vi "Autonomous Independent.vi"() -> ()   [LabVIEW 2016]
doc: "This VI is called when autonomous begins, and will automatically be terminated when autonomous ends. You can carry out timed or sensor driven robot movement independently without needing to return to the caller."
uses:
  <vilib>/Rock Robotics/WPI/Utilities/WPI_GetSetVariantRefNum.vi
  <vilib>/Rock Robotics/WPI/RobotDrive/WPI_RobotDriveArcadeDrive_Standard(NoSaturation).vi
  <vilib>/Rock Robotics/Network Tables/SD Read Number.vi
  <vilib>/Rock Robotics/WPI/Solenoid/Deprecated/WPI_SolenoidSetBool.vi
panel:
  out "Current Movement, for debugging":T1 {"Y Joystick Value" scale=1.0..-1.0; "X Joystick Value" scale=-1.0..1.0}
  in  "Array of robot movements":T2(array[cluster]) {"Y Joystick Value" scale=1.0..-1.0; "X Joystick Value" scale=-1.0..1.0}
  # "Be sure to right-click and choose Data Operations>>Make Current Value default if you want to save the array values with the VI"
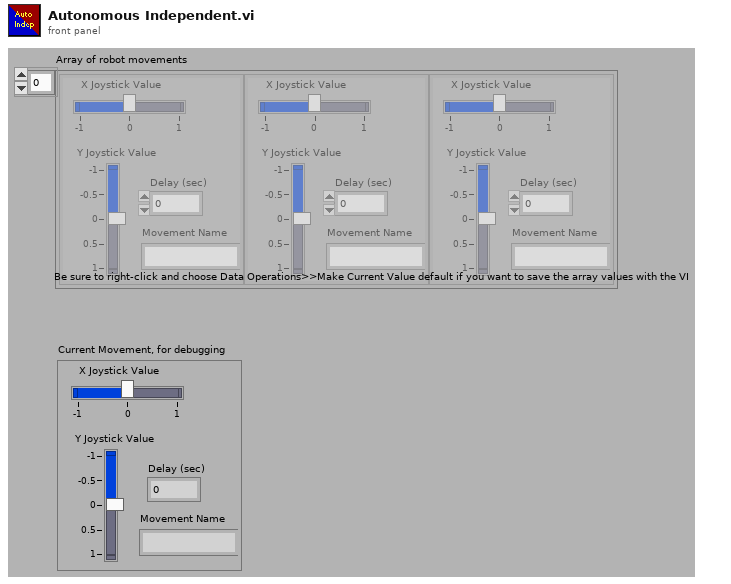
[diagram p1: front panel]
types:
  T1 = cluster{"X Joystick Value":dbl, "Y Joystick Value":dbl, "Delay (sec)":dbl, "Movement Name":string}
  T2 = cluster{"X Joystick Value":dbl, "Y Joystick Value":dbl, "Delay (sec)":dbl, "Movement Name":string}[]
  T3 = typedef "WPI_MotorControlDeviceRef.ctl" = cluster{"DeviceStatus":errorcluster, "Type":T4, "PWM":cluster{"PWM Channel":T5, "DeadBand":T6}, "CAN":cluster{"Device Number":u8, "SetOutput VI Ref":variant, "GetOutput VI Ref":variant, "Enable VI Ref":variant, "Disable VI Ref":variant, "Data":variant}, "Invert":bool}
  T4 = typedef "WPI_MotorControlType.ctl" = enum16{"PWM", "CAN"}
  T5 = typedef "FPGA_DIOPWMChannel.ctl" = enum8{"PWM 0", "PWM 1", "PWM 2", "PWM 3", "PWM 4", "PWM 5", "PWM 6", "PWM 7", "PWM 8", "PWM 9", "PWM MXP 0", "PWM MXP 1", "PWM MXP 2", "PWM MXP 3", "PWM MXP 4", "PWM MXP 5", "PWM MXP 6", "PWM MXP 7", "PWM MXP 8", "PWM MXP 9", "Invalid"}
  T6 = typedef "WPI_PWMDeadband.ctl" = cluster{"Name":string, "maxPositivePwm":i32, "minPositivePwm":i32, "centerPwm":i32, "maxNegativePwm":i32, "minNegativePwm":i32, "angularRange":u16}
  T7 = typedef "WPI_SolenoidDevRef.ctl" = cluster{"DevStatus":errorcluster, "Pneumatics Control Module":u8, "Forward Solenoid Channel":T8, "Reverse Solenoid Channel":T8}
  T8 = typedef "WPI_SolenoidChannel.ctl" = enum8{"Solenoid 0", "Solenoid 1", "Solenoid 2", "Solenoid 3", "Solenoid 4", "Solenoid 5", "Solenoid 6", "Solenoid 7", "Invalid"}
  T9 = typedef "WPI_RobotDriveDevRef.ctl" = cluster{"DevStatus":errorcluster, "Motors[]":T3[], "Square Inputs":bool, "Max Output":dbl}
  T10 = typedef "WPI_JoystickDevRef.ctl" = cluster{"Device":T11}
  T11 = typedef "WPI_JoystickDeviceEnum.ctl" = enum16{"USB 0", "USB 1", "USB 2", "USB 3", "USB 4", "USB 5"}
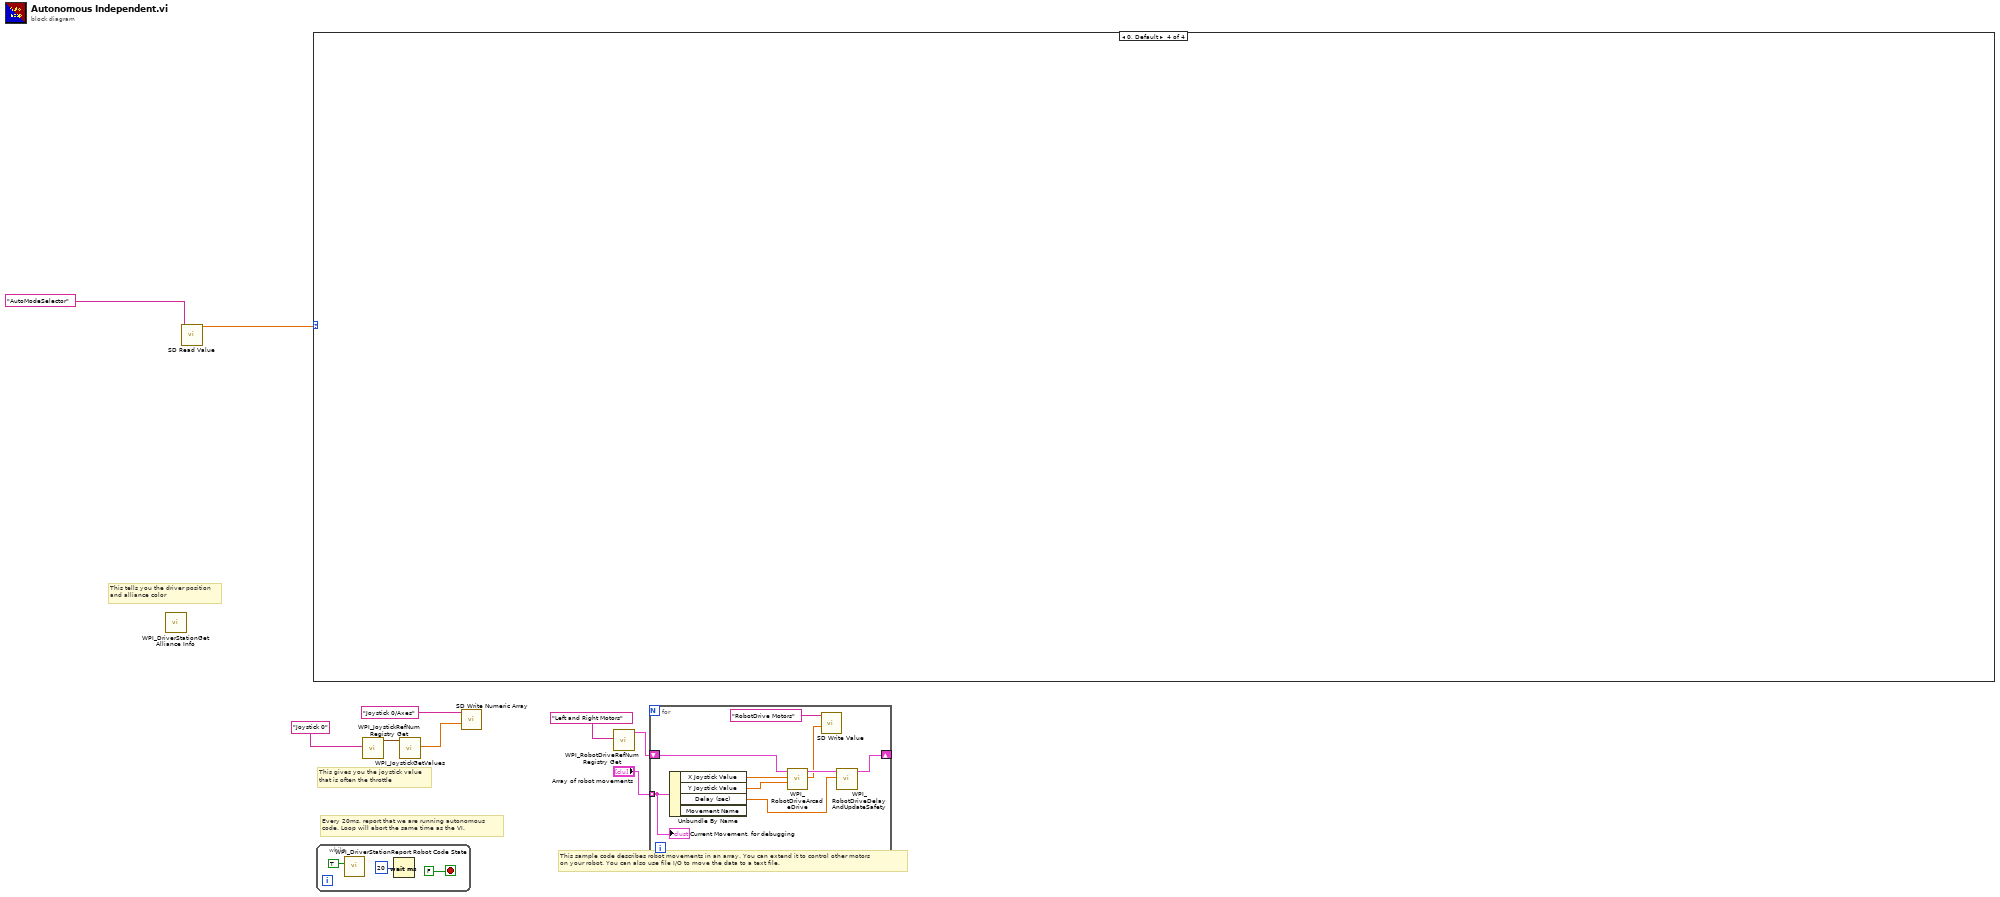
[diagram p0: block diagram]
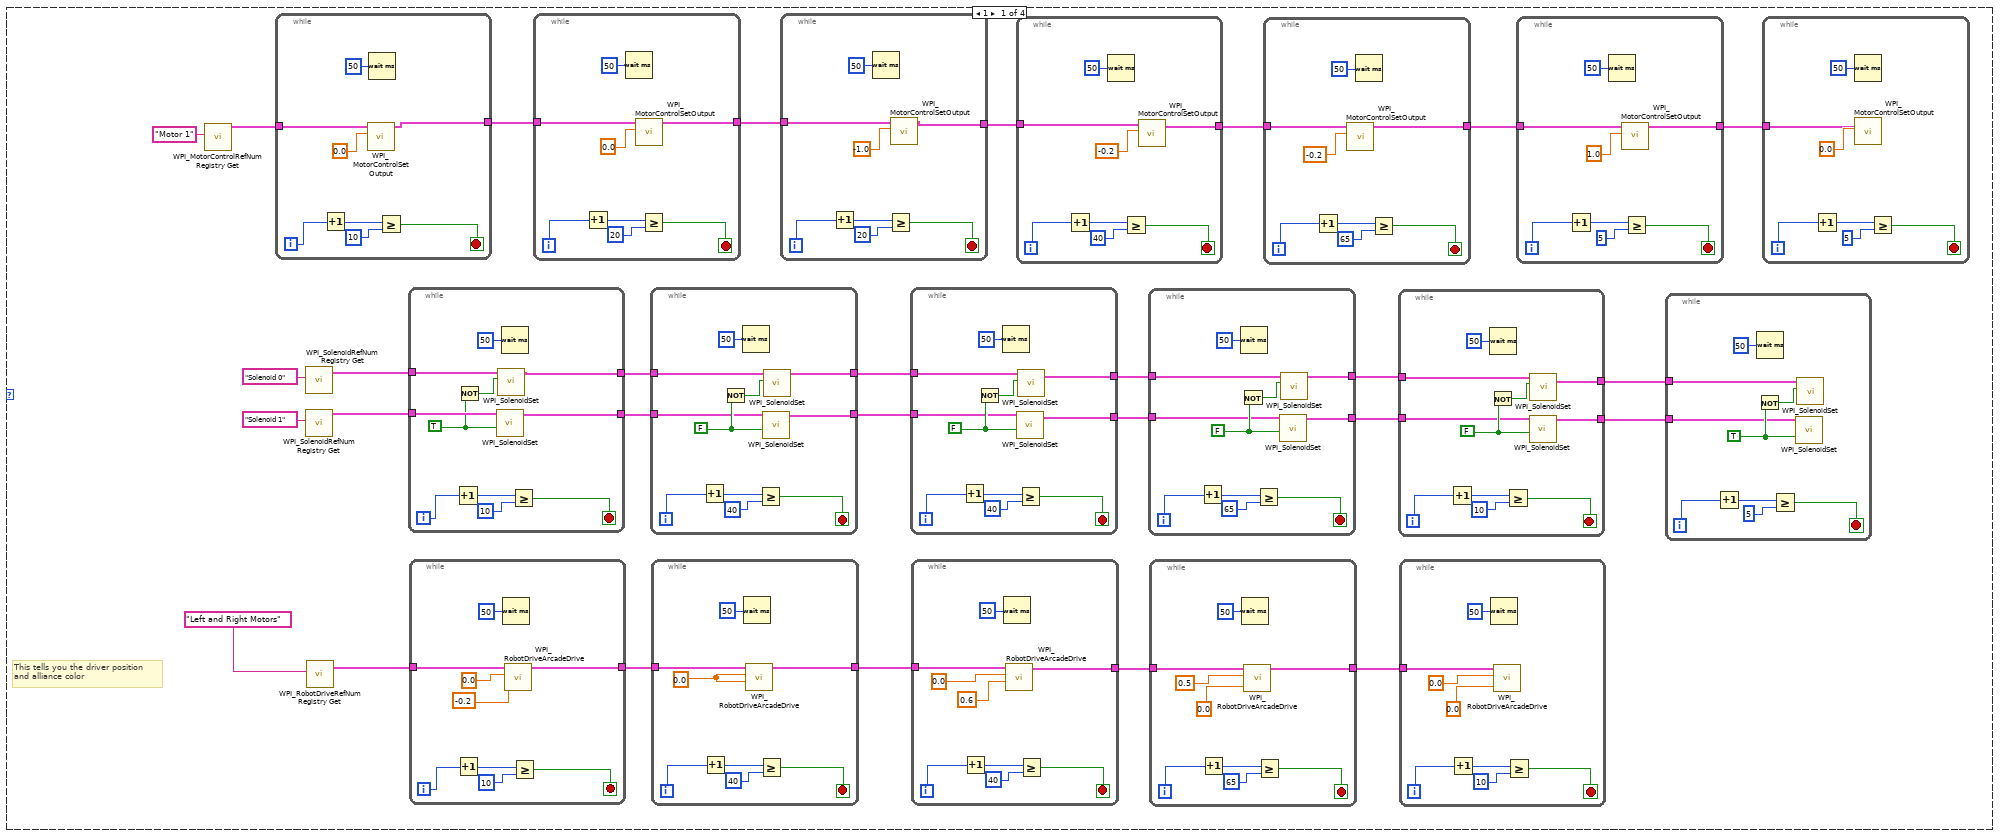
[diagram p2: hidden frame]
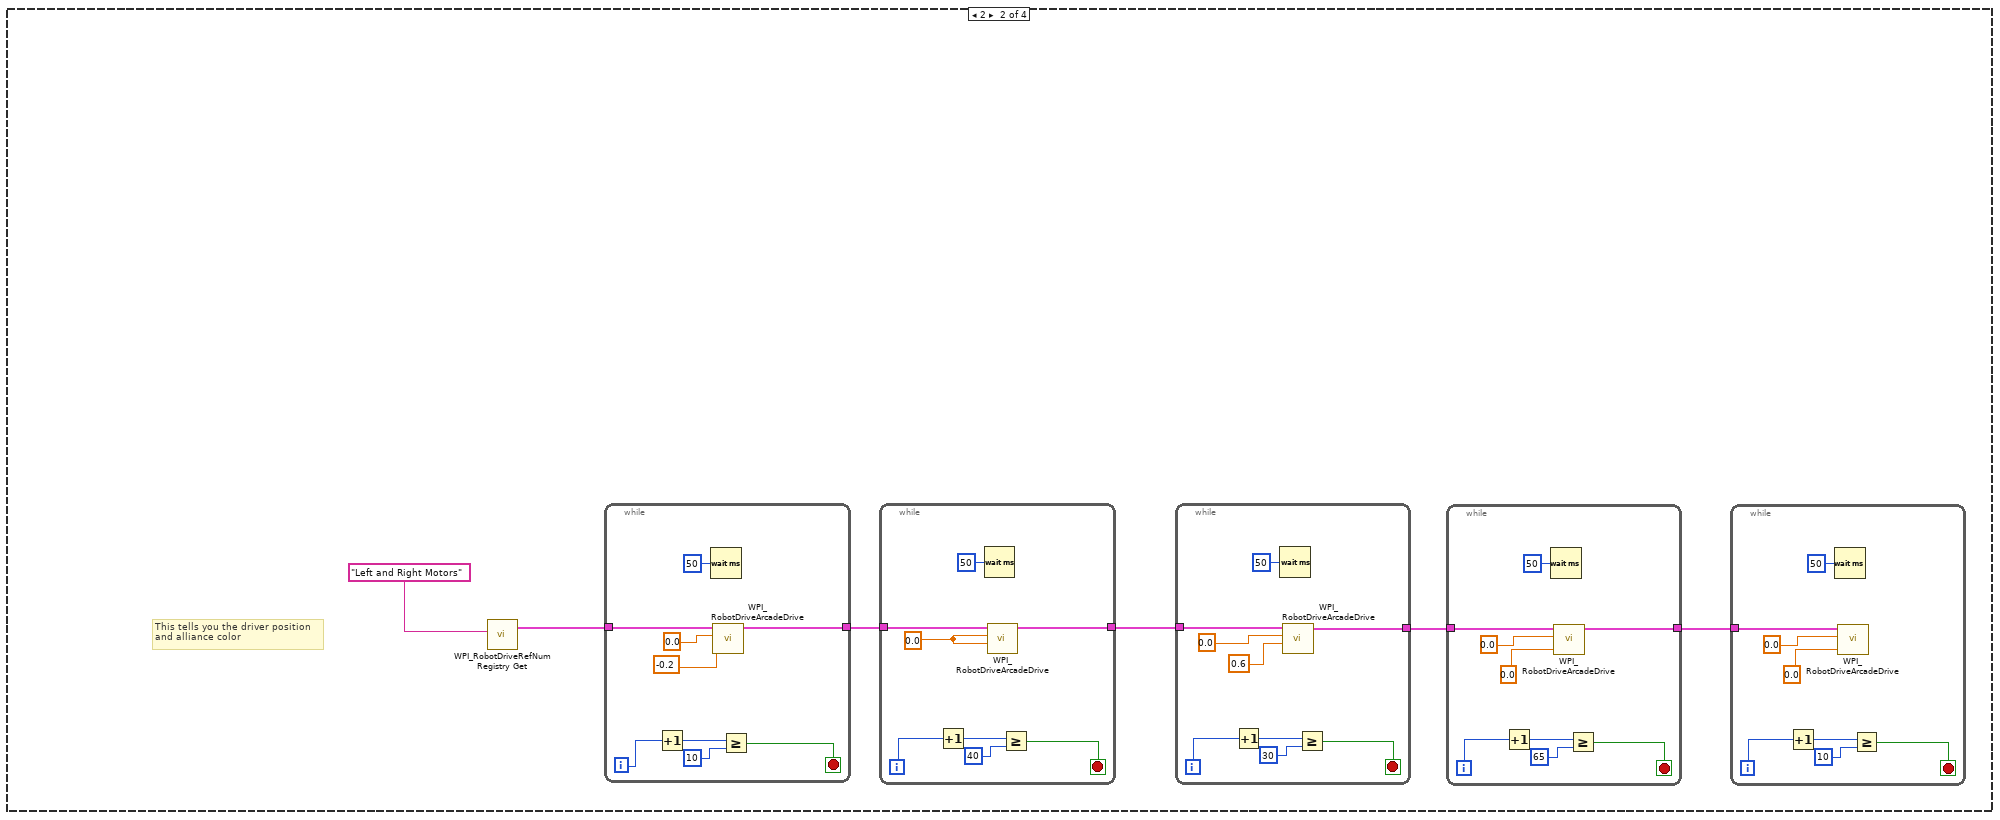
[diagram p3: hidden frame]
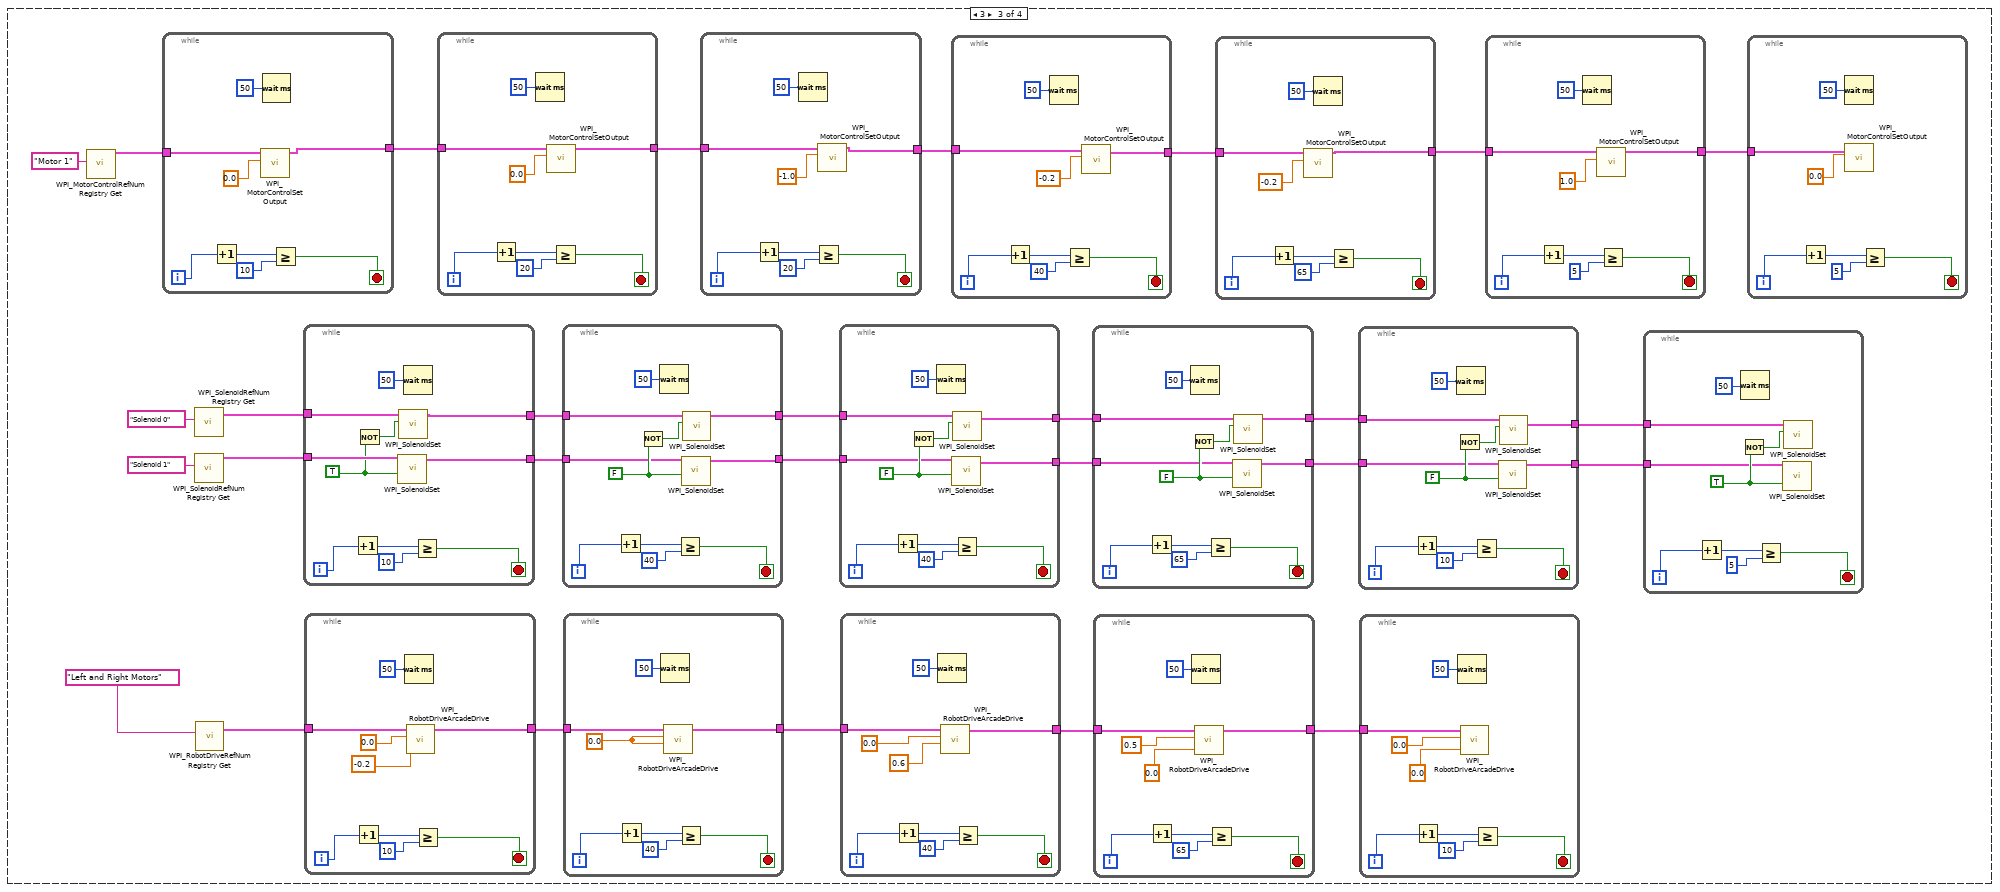
[diagram p4: hidden frame]
diagram:
  # "This tells you the driver position\nand alliance color"
  # "This sample code describes robot movements in an array. You can extend it to control other motors\non your robot. You can also use file I/O to move the data to a text file."
  # "Every 20ms, report that we are running autonomous\ncode. Loop will abort the same time as the VI."
  # "This gives you the joystick value\nthat is often the throttle"
  n1 = call <vilib>:"WPI_DriverStationGet Alliance Info.vi"() -> ()  [unwired: 12 out]
  n2 = call-poly <vilib>:"SD Read Value.vi"("Name"="AutoModeSelector") -> ("Numeric"=w2:dbl)  [unwired: 8 in, 2 out]
  n3 = case shown="0, Default" w2 {
    frame 1 {
      # "This tells you the driver position\nand alliance color"
      n4 = call <vilib>:"WPI_MotorControlRefNum Registry Get.vi"("refnum name"="Motor 1") -> ("MotorControlDevRef"=w18:T3)  [unwired: 9 in, 1 out]
      n5 = while {
        tunnel: w18 -> [w115]
        tunnel: [w113] -> w17
        i -> [w120]
        stop <- w116 stop-if-true
        n6 = Increment(x=w120) -> (x+1=w119:i32)
        n7 = call <vilib>:"WPI_MotorControlSetOutput.vi"("Output"=0.0, "MotorControlDevRef"=w115) -> ("MotorControlDevRef"=w113:T3)  [unwired: 7 in, 2 out]
        n8 = Wait (ms)(milliseconds to wait=u32 50) -> ()  [unwired: 1 out]
        n9 = Greater Or Equal?(x=w119, y=10) -> (x >= y?=w116:bool)
      }
      n10 = call <vilib>:"WPI_SolenoidRefNum Registry Get.vi"("refnum name"="Solenoid 0") -> ("SolenoidDevRef"=w30:T7)  [unwired: 9 in, 1 out]
      n11 = call <vilib>:"WPI_SolenoidRefNum Registry Get.vi"("refnum name"="Solenoid 1") -> ("SolenoidDevRef"=w29:T7)  [unwired: 9 in, 1 out]
      n12 = call <vilib>:"WPI_RobotDriveRefNum Registry Get.vi"("refnum name"="Left and Right Motors") -> ("RobotDriveDevRef"=w36:T9)  [unwired: 9 in, 1 out]
      n13 = while {
        tunnel: w30 -> [w159]
        tunnel: w29 -> [w158]
        tunnel: [w155] -> w28
        tunnel: [w154] -> w27
        i -> [w164]
        stop <- w160 stop-if-true
        w157 = TRUE
        n14 = Increment(x=w164) -> (x+1=w163:i32)
        n15 = Not(x=w157) -> (.not. x?=w156:bool)
        n16 = call-poly <vilib>:"WPI_SolenoidSet.vi"("Value"=w157, "SolenoidDevRef"=w158) -> ("SolenoidDevRef"=w154:T7)  [unwired: 8 in, 1 out]
        n17 = call-poly <vilib>:"WPI_SolenoidSet.vi"("Value"=w156, "SolenoidDevRef"=w159) -> ("SolenoidDevRef"=w155:T7)  [unwired: 8 in, 1 out]
        n18 = Wait (ms)(milliseconds to wait=u32 50) -> ()  [unwired: 1 out]
        n19 = Greater Or Equal?(x=w163, y=10) -> (x >= y?=w160:bool)
      }
      n20 = while {
        tunnel: w36 -> [w199]
        tunnel: [w192] -> w35
        i -> [w197]
        stop <- w193 stop-if-true
        n21 = Increment(x=w197) -> (x+1=w196:i32)
        n22 = Wait (ms)(milliseconds to wait=u32 50) -> ()  [unwired: 1 out]
        n23 = call-poly <vilib>:"WPI_RobotDriveArcadeDrive.vi"("Y axis value"=-0.2, "X axis value"=0.0, "RobotDriveDevRef"=w199) -> ("RobotDriveDevRef"=w192:T9)  [unwired: 6 in, 2 out]
        n24 = Greater Or Equal?(x=w196, y=10) -> (x >= y?=w193:bool)
      }
      n25 = while {
        tunnel: w17 -> [w106]
        tunnel: [w105] -> w16
        i -> [w108]
        stop <- w109 stop-if-true
        n26 = Increment(x=w108) -> (x+1=w111:i32)
        n27 = Wait (ms)(milliseconds to wait=u32 50) -> ()  [unwired: 1 out]
        n28 = call <vilib>:"WPI_MotorControlSetOutput.vi"("Output"=0.0, "MotorControlDevRef"=w106) -> ("MotorControlDevRef"=w105:T3)  [unwired: 7 in, 2 out]
        n29 = Greater Or Equal?(x=w111, y=20) -> (x >= y?=w109:bool)
      }
      n30 = while {
        tunnel: w28 -> [w146]
        tunnel: w27 -> [w145]
        tunnel: [w144] -> w26
        tunnel: [w143] -> w25
        i -> [w149]
        stop <- w150 stop-if-true
        w148 = FALSE
        n31 = Increment(x=w149) -> (x+1=w152:i32)
        n32 = Not(x=w148) -> (.not. x?=w147:bool)
        n33 = Wait (ms)(milliseconds to wait=u32 50) -> ()  [unwired: 1 out]
        n34 = Greater Or Equal?(x=w152, y=40) -> (x >= y?=w150:bool)
        n35 = call-poly <vilib>:"WPI_SolenoidSet.vi"("Value"=w148, "SolenoidDevRef"=w145) -> ("SolenoidDevRef"=w143:T7)  [unwired: 8 in, 1 out]
        n36 = call-poly <vilib>:"WPI_SolenoidSet.vi"("Value"=w147, "SolenoidDevRef"=w146) -> ("SolenoidDevRef"=w144:T7)  [unwired: 8 in, 1 out]
      }
      n37 = while {
        tunnel: w35 -> [w190]
        tunnel: [w183] -> w34
        i -> [w184]
        stop <- w185 stop-if-true
        w189 = 0.0 ("X axis value")
        n38 = Increment(x=w184) -> (x+1=w187:i32)
        n39 = Wait (ms)(milliseconds to wait=u32 50) -> ()  [unwired: 1 out]
        n40 = call-poly <vilib>:"WPI_RobotDriveArcadeDrive.vi"("Y axis value"=w189, "X axis value"=w189, "RobotDriveDevRef"=w190) -> ("RobotDriveDevRef"=w183:T9)  [unwired: 6 in, 2 out]
        n41 = Greater Or Equal?(x=w187, y=40) -> (x >= y?=w185:bool)
      }
      n42 = while {
        tunnel: w16 -> [w98]
        tunnel: [w97] -> w15
        i -> [w100]
        stop <- w101 stop-if-true
        n43 = Increment(x=w100) -> (x+1=w103:i32)
        n44 = Wait (ms)(milliseconds to wait=u32 50) -> ()  [unwired: 1 out]
        n45 = Greater Or Equal?(x=w103, y=20) -> (x >= y?=w101:bool)
        n46 = call <vilib>:"WPI_MotorControlSetOutput.vi"("Output"=-1.0, "MotorControlDevRef"=w98) -> ("MotorControlDevRef"=w97:T3)  [unwired: 7 in, 2 out]
      }
      n47 = while {
        tunnel: w26 -> [w135]
        tunnel: w25 -> [w134]
        tunnel: [w133] -> w23
        tunnel: [w132] -> w22
        i -> [w138]
        stop <- w139 stop-if-true
        w137 = FALSE
        n48 = Increment(x=w138) -> (x+1=w141:i32)
        n49 = Not(x=w137) -> (.not. x?=w136:bool)
        n50 = Wait (ms)(milliseconds to wait=u32 50) -> ()  [unwired: 1 out]
        n51 = call-poly <vilib>:"WPI_SolenoidSet.vi"("Value"=w137, "SolenoidDevRef"=w134) -> ("SolenoidDevRef"=w132:T7)  [unwired: 8 in, 1 out]
        n52 = call-poly <vilib>:"WPI_SolenoidSet.vi"("Value"=w136, "SolenoidDevRef"=w135) -> ("SolenoidDevRef"=w133:T7)  [unwired: 8 in, 1 out]
        n53 = Greater Or Equal?(x=w141, y=40) -> (x >= y?=w139:bool)
      }
      n54 = while {
        tunnel: w34 -> [w182]
        tunnel: [w174] -> w33
        i -> [w177]
        stop <- w178 stop-if-true
        n55 = Increment(x=w177) -> (x+1=w180:i32)
        n56 = Wait (ms)(milliseconds to wait=u32 50) -> ()  [unwired: 1 out]
        n57 = call-poly <vilib>:"WPI_RobotDriveArcadeDrive.vi"("Y axis value"=0.6, "X axis value"=0.0, "RobotDriveDevRef"=w182) -> ("RobotDriveDevRef"=w174:T9)  [unwired: 6 in, 2 out]
        n58 = Greater Or Equal?(x=w180, y=40) -> (x >= y?=w178:bool)
      }
      n59 = while {
        tunnel: w15 -> [w90]
        tunnel: [w89] -> w14
        i -> [w92]
        stop <- w93 stop-if-true
        n60 = Increment(x=w92) -> (x+1=w95:i32)
        n61 = Wait (ms)(milliseconds to wait=u32 50) -> ()  [unwired: 1 out]
        n62 = Greater Or Equal?(x=w95, y=40) -> (x >= y?=w93:bool)
        n63 = call <vilib>:"WPI_MotorControlSetOutput.vi"("Output"=-0.2, "MotorControlDevRef"=w90) -> ("MotorControlDevRef"=w89:T3)  [unwired: 7 in, 2 out]
      }
      n64 = while {
        tunnel: w23 -> [w124]
        tunnel: w22 -> [w123]
        tunnel: [w122] -> w21
        tunnel: [w121] -> w20
        i -> [w127]
        stop <- w128 stop-if-true
        w126 = FALSE
        n65 = Increment(x=w127) -> (x+1=w130:i32)
        n66 = Not(x=w126) -> (.not. x?=w125:bool)
        n67 = Wait (ms)(milliseconds to wait=u32 50) -> ()  [unwired: 1 out]
        n68 = Greater Or Equal?(x=w130, y=65) -> (x >= y?=w128:bool)
        n69 = call-poly <vilib>:"WPI_SolenoidSet.vi"("Value"=w126, "SolenoidDevRef"=w123) -> ("SolenoidDevRef"=w121:T7)  [unwired: 8 in, 1 out]
        n70 = call-poly <vilib>:"WPI_SolenoidSet.vi"("Value"=w125, "SolenoidDevRef"=w124) -> ("SolenoidDevRef"=w122:T7)  [unwired: 8 in, 1 out]
      }
      n71 = while {
        tunnel: w33 -> [w173]
        tunnel: [w165] -> w24
        i -> [w167]
        stop <- w168 stop-if-true
        n72 = Increment(x=w167) -> (x+1=w170:i32)
        n73 = Wait (ms)(milliseconds to wait=u32 50) -> ()  [unwired: 1 out]
        n74 = call-poly <vilib>:"WPI_RobotDriveArcadeDrive.vi"("Y axis value"=0.0 ("X axis value"), "X axis value"=0.5, "RobotDriveDevRef"=w173) -> ("RobotDriveDevRef"=w165:T9)  [unwired: 6 in, 2 out]
        n75 = Greater Or Equal?(x=w170, y=65) -> (x >= y?=w168:bool)
      }
      n76 = while {
        tunnel: w14 -> [w63]
        tunnel: [w62] -> w13
        i -> [w65]
        stop <- w66 stop-if-true
        n77 = Increment(x=w65) -> (x+1=w68:i32)
        n78 = call <vilib>:"WPI_MotorControlSetOutput.vi"("Output"=-0.2, "MotorControlDevRef"=w63) -> ("MotorControlDevRef"=w62:T3)  [unwired: 7 in, 2 out]
        n79 = Wait (ms)(milliseconds to wait=u32 50) -> ()  [unwired: 1 out]
        n80 = Greater Or Equal?(x=w68, y=65) -> (x >= y?=w66:bool)
      }
      n81 = while {
        tunnel: w21 -> [w73]
        tunnel: w20 -> [w72]
        tunnel: [w71] -> w11
        tunnel: [w70] -> w10
        i -> [w76]
        stop <- w77 stop-if-true
        w75 = FALSE
        n82 = Increment(x=w76) -> (x+1=w79:i32)
        n83 = Not(x=w75) -> (.not. x?=w74:bool)
        n84 = Wait (ms)(milliseconds to wait=u32 50) -> ()  [unwired: 1 out]
        n85 = Greater Or Equal?(x=w79, y=10) -> (x >= y?=w77:bool)
        n86 = call-poly <vilib>:"WPI_SolenoidSet.vi"("Value"=w75, "SolenoidDevRef"=w72) -> ("SolenoidDevRef"=w70:T7)  [unwired: 8 in, 1 out]
        n87 = call-poly <vilib>:"WPI_SolenoidSet.vi"("Value"=w74, "SolenoidDevRef"=w73) -> ("SolenoidDevRef"=w71:T7)  [unwired: 8 in, 1 out]
      }
      n88 = while {
        tunnel: w24 -> [w88]
        i -> [w82]
        stop <- w83 stop-if-true
        n89 = Increment(x=w82) -> (x+1=w85:i32)
        n90 = Wait (ms)(milliseconds to wait=u32 50) -> ()  [unwired: 1 out]
        n91 = call-poly <vilib>:"WPI_RobotDriveArcadeDrive.vi"("Y axis value"=0.0 ("X axis value"), "X axis value"=0.0, "RobotDriveDevRef"=w88) -> ()  [unwired: 6 in, 3 out]
        n92 = Greater Or Equal?(x=w85, y=10) -> (x >= y?=w83:bool)
      }
      n93 = while {
        tunnel: w13 -> [w55]
        tunnel: [w54] -> w12
        i -> [w57]
        stop <- w58 stop-if-true
        n94 = Increment(x=w57) -> (x+1=w60:i32)
        n95 = Wait (ms)(milliseconds to wait=u32 50) -> ()  [unwired: 1 out]
        n96 = call <vilib>:"WPI_MotorControlSetOutput.vi"("Output"=1.0, "MotorControlDevRef"=w55) -> ("MotorControlDevRef"=w54:T3)  [unwired: 7 in, 2 out]
        n97 = Greater Or Equal?(x=w60, y=5) -> (x >= y?=w58:bool)
      }
      n98 = while {
        tunnel: w11 -> [w39]
        tunnel: w10 -> [w38]
        i -> [w42]
        stop <- w43 stop-if-true
        w41 = TRUE
        n99 = Increment(x=w42) -> (x+1=w45:i32)
        n100 = Not(x=w41) -> (.not. x?=w40:bool)
        n101 = Wait (ms)(milliseconds to wait=u32 50) -> ()  [unwired: 1 out]
        n102 = Greater Or Equal?(x=w45, y=5) -> (x >= y?=w43:bool)
        n103 = call-poly <vilib>:"WPI_SolenoidSet.vi"("Value"=w41, "SolenoidDevRef"=w38) -> ()  [unwired: 8 in, 2 out]
        n104 = call-poly <vilib>:"WPI_SolenoidSet.vi"("Value"=w40, "SolenoidDevRef"=w39) -> ()  [unwired: 8 in, 2 out]
      }
      n105 = while {
        tunnel: w12 -> [w47]
        i -> [w49]
        stop <- w50 stop-if-true
        n106 = Increment(x=w49) -> (x+1=w52:i32)
        n107 = Wait (ms)(milliseconds to wait=u32 50) -> ()  [unwired: 1 out]
        n108 = call <vilib>:"WPI_MotorControlSetOutput.vi"("Output"=0.0, "MotorControlDevRef"=w47) -> ()  [unwired: 7 in, 3 out]
        n109 = Greater Or Equal?(x=w52, y=5) -> (x >= y?=w50:bool)
      }
    }
    frame 2 {
      # "This tells you the driver position\nand alliance color"
      n110 = call <vilib>:"WPI_RobotDriveRefNum Registry Get.vi"("refnum name"="Left and Right Motors") -> ("RobotDriveDevRef"=w204:T9)  [unwired: 9 in, 1 out]
      n111 = while {
        tunnel: w204 -> [w248]
        tunnel: [w241] -> w203
        i -> [w246]
        stop <- w242 stop-if-true
        n112 = Increment(x=w246) -> (x+1=w245:i32)
        n113 = Wait (ms)(milliseconds to wait=u32 50) -> ()  [unwired: 1 out]
        n114 = call-poly <vilib>:"WPI_RobotDriveArcadeDrive.vi"("Y axis value"=-0.2, "X axis value"=0.0, "RobotDriveDevRef"=w248) -> ("RobotDriveDevRef"=w241:T9)  [unwired: 6 in, 2 out]
        n115 = Greater Or Equal?(x=w245, y=10) -> (x >= y?=w242:bool)
      }
      n116 = while {
        tunnel: w203 -> [w239]
        tunnel: [w232] -> w202
        i -> [w233]
        stop <- w234 stop-if-true
        w238 = 0.0 ("X axis value")
        n117 = Increment(x=w233) -> (x+1=w236:i32)
        n118 = Wait (ms)(milliseconds to wait=u32 50) -> ()  [unwired: 1 out]
        n119 = call-poly <vilib>:"WPI_RobotDriveArcadeDrive.vi"("Y axis value"=w238, "X axis value"=w238, "RobotDriveDevRef"=w239) -> ("RobotDriveDevRef"=w232:T9)  [unwired: 6 in, 2 out]
        n120 = Greater Or Equal?(x=w236, y=40) -> (x >= y?=w234:bool)
      }
      n121 = while {
        tunnel: w202 -> [w231]
        tunnel: [w223] -> w201
        i -> [w226]
        stop <- w227 stop-if-true
        n122 = Increment(x=w226) -> (x+1=w229:i32)
        n123 = Wait (ms)(milliseconds to wait=u32 50) -> ()  [unwired: 1 out]
        n124 = call-poly <vilib>:"WPI_RobotDriveArcadeDrive.vi"("Y axis value"=0.6, "X axis value"=0.0, "RobotDriveDevRef"=w231) -> ("RobotDriveDevRef"=w223:T9)  [unwired: 6 in, 2 out]
        n125 = Greater Or Equal?(x=w229, y=30) -> (x >= y?=w227:bool)
      }
      n126 = while {
        tunnel: w201 -> [w222]
        tunnel: [w214] -> w200
        i -> [w216]
        stop <- w217 stop-if-true
        n127 = Increment(x=w216) -> (x+1=w219:i32)
        n128 = Wait (ms)(milliseconds to wait=u32 50) -> ()  [unwired: 1 out]
        n129 = call-poly <vilib>:"WPI_RobotDriveArcadeDrive.vi"("Y axis value"=0.0 ("X axis value"), "X axis value"=0.0, "RobotDriveDevRef"=w222) -> ("RobotDriveDevRef"=w214:T9)  [unwired: 6 in, 2 out]
        n130 = Greater Or Equal?(x=w219, y=65) -> (x >= y?=w217:bool)
      }
      n131 = while {
        tunnel: w200 -> [w213]
        i -> [w207]
        stop <- w208 stop-if-true
        n132 = Increment(x=w207) -> (x+1=w210:i32)
        n133 = Wait (ms)(milliseconds to wait=u32 50) -> ()  [unwired: 1 out]
        n134 = call-poly <vilib>:"WPI_RobotDriveArcadeDrive.vi"("Y axis value"=0.0 ("X axis value"), "X axis value"=0.0, "RobotDriveDevRef"=w213) -> ()  [unwired: 6 in, 3 out]
        n135 = Greater Or Equal?(x=w210, y=10) -> (x >= y?=w208:bool)
      }
    }
    frame 3 {
      n136 = call <vilib>:"WPI_MotorControlRefNum Registry Get.vi"("refnum name"="Motor 1") -> ("MotorControlDevRef"=w257:T3)  [unwired: 9 in, 1 out]
      n137 = while {
        tunnel: w257 -> [w354]
        tunnel: [w352] -> w256
        i -> [w359]
        stop <- w355 stop-if-true
        n138 = Increment(x=w359) -> (x+1=w358:i32)
        n139 = call <vilib>:"WPI_MotorControlSetOutput.vi"("Output"=0.0, "MotorControlDevRef"=w354) -> ("MotorControlDevRef"=w352:T3)  [unwired: 7 in, 2 out]
        n140 = Wait (ms)(milliseconds to wait=u32 50) -> ()  [unwired: 1 out]
        n141 = Greater Or Equal?(x=w358, y=10) -> (x >= y?=w355:bool)
      }
      n142 = call <vilib>:"WPI_SolenoidRefNum Registry Get.vi"("refnum name"="Solenoid 0") -> ("SolenoidDevRef"=w269:T7)  [unwired: 9 in, 1 out]
      n143 = call <vilib>:"WPI_SolenoidRefNum Registry Get.vi"("refnum name"="Solenoid 1") -> ("SolenoidDevRef"=w268:T7)  [unwired: 9 in, 1 out]
      n144 = call <vilib>:"WPI_RobotDriveRefNum Registry Get.vi"("refnum name"="Left and Right Motors") -> ("RobotDriveDevRef"=w275:T9)  [unwired: 9 in, 1 out]
      n145 = while {
        tunnel: w269 -> [w398]
        tunnel: w268 -> [w397]
        tunnel: [w394] -> w267
        tunnel: [w393] -> w266
        i -> [w403]
        stop <- w399 stop-if-true
        w396 = TRUE
        n146 = Increment(x=w403) -> (x+1=w402:i32)
        n147 = Not(x=w396) -> (.not. x?=w395:bool)
        n148 = call-poly <vilib>:"WPI_SolenoidSet.vi"("Value"=w396, "SolenoidDevRef"=w397) -> ("SolenoidDevRef"=w393:T7)  [unwired: 8 in, 1 out]
        n149 = call-poly <vilib>:"WPI_SolenoidSet.vi"("Value"=w395, "SolenoidDevRef"=w398) -> ("SolenoidDevRef"=w394:T7)  [unwired: 8 in, 1 out]
        n150 = Wait (ms)(milliseconds to wait=u32 50) -> ()  [unwired: 1 out]
        n151 = Greater Or Equal?(x=w402, y=10) -> (x >= y?=w399:bool)
      }
      n152 = while {
        tunnel: w275 -> [w438]
        tunnel: [w431] -> w274
        i -> [w436]
        stop <- w432 stop-if-true
        n153 = Increment(x=w436) -> (x+1=w435:i32)
        n154 = Wait (ms)(milliseconds to wait=u32 50) -> ()  [unwired: 1 out]
        n155 = call-poly <vilib>:"WPI_RobotDriveArcadeDrive.vi"("Y axis value"=-0.2, "X axis value"=0.0, "RobotDriveDevRef"=w438) -> ("RobotDriveDevRef"=w431:T9)  [unwired: 6 in, 2 out]
        n156 = Greater Or Equal?(x=w435, y=10) -> (x >= y?=w432:bool)
      }
      n157 = while {
        tunnel: w256 -> [w345]
        tunnel: [w344] -> w255
        i -> [w347]
        stop <- w348 stop-if-true
        n158 = Increment(x=w347) -> (x+1=w350:i32)
        n159 = Wait (ms)(milliseconds to wait=u32 50) -> ()  [unwired: 1 out]
        n160 = call <vilib>:"WPI_MotorControlSetOutput.vi"("Output"=0.0, "MotorControlDevRef"=w345) -> ("MotorControlDevRef"=w344:T3)  [unwired: 7 in, 2 out]
        n161 = Greater Or Equal?(x=w350, y=20) -> (x >= y?=w348:bool)
      }
      n162 = while {
        tunnel: w267 -> [w385]
        tunnel: w266 -> [w384]
        tunnel: [w383] -> w265
        tunnel: [w382] -> w264
        i -> [w388]
        stop <- w389 stop-if-true
        w387 = FALSE
        n163 = Increment(x=w388) -> (x+1=w391:i32)
        n164 = Not(x=w387) -> (.not. x?=w386:bool)
        n165 = Wait (ms)(milliseconds to wait=u32 50) -> ()  [unwired: 1 out]
        n166 = Greater Or Equal?(x=w391, y=40) -> (x >= y?=w389:bool)
        n167 = call-poly <vilib>:"WPI_SolenoidSet.vi"("Value"=w387, "SolenoidDevRef"=w384) -> ("SolenoidDevRef"=w382:T7)  [unwired: 8 in, 1 out]
        n168 = call-poly <vilib>:"WPI_SolenoidSet.vi"("Value"=w386, "SolenoidDevRef"=w385) -> ("SolenoidDevRef"=w383:T7)  [unwired: 8 in, 1 out]
      }
      n169 = while {
        tunnel: w274 -> [w429]
        tunnel: [w422] -> w273
        i -> [w423]
        stop <- w424 stop-if-true
        w428 = 0.0 ("X axis value")
        n170 = Increment(x=w423) -> (x+1=w426:i32)
        n171 = Wait (ms)(milliseconds to wait=u32 50) -> ()  [unwired: 1 out]
        n172 = call-poly <vilib>:"WPI_RobotDriveArcadeDrive.vi"("Y axis value"=w428, "X axis value"=w428, "RobotDriveDevRef"=w429) -> ("RobotDriveDevRef"=w422:T9)  [unwired: 6 in, 2 out]
        n173 = Greater Or Equal?(x=w426, y=40) -> (x >= y?=w424:bool)
      }
      n174 = while {
        tunnel: w255 -> [w337]
        tunnel: [w336] -> w254
        i -> [w339]
        stop <- w340 stop-if-true
        n175 = Increment(x=w339) -> (x+1=w342:i32)
        n176 = Wait (ms)(milliseconds to wait=u32 50) -> ()  [unwired: 1 out]
        n177 = Greater Or Equal?(x=w342, y=20) -> (x >= y?=w340:bool)
        n178 = call <vilib>:"WPI_MotorControlSetOutput.vi"("Output"=-1.0, "MotorControlDevRef"=w337) -> ("MotorControlDevRef"=w336:T3)  [unwired: 7 in, 2 out]
      }
      n179 = while {
        tunnel: w265 -> [w374]
        tunnel: w264 -> [w373]
        tunnel: [w372] -> w262
        tunnel: [w371] -> w261
        i -> [w377]
        stop <- w378 stop-if-true
        w376 = FALSE
        n180 = Increment(x=w377) -> (x+1=w380:i32)
        n181 = Not(x=w376) -> (.not. x?=w375:bool)
        n182 = Wait (ms)(milliseconds to wait=u32 50) -> ()  [unwired: 1 out]
        n183 = call-poly <vilib>:"WPI_SolenoidSet.vi"("Value"=w376, "SolenoidDevRef"=w373) -> ("SolenoidDevRef"=w371:T7)  [unwired: 8 in, 1 out]
        n184 = call-poly <vilib>:"WPI_SolenoidSet.vi"("Value"=w375, "SolenoidDevRef"=w374) -> ("SolenoidDevRef"=w372:T7)  [unwired: 8 in, 1 out]
        n185 = Greater Or Equal?(x=w380, y=40) -> (x >= y?=w378:bool)
      }
      n186 = while {
        tunnel: w273 -> [w421]
        tunnel: [w413] -> w272
        i -> [w416]
        stop <- w417 stop-if-true
        n187 = Increment(x=w416) -> (x+1=w419:i32)
        n188 = Wait (ms)(milliseconds to wait=u32 50) -> ()  [unwired: 1 out]
        n189 = call-poly <vilib>:"WPI_RobotDriveArcadeDrive.vi"("Y axis value"=0.6, "X axis value"=0.0, "RobotDriveDevRef"=w421) -> ("RobotDriveDevRef"=w413:T9)  [unwired: 6 in, 2 out]
        n190 = Greater Or Equal?(x=w419, y=40) -> (x >= y?=w417:bool)
      }
      n191 = while {
        tunnel: w254 -> [w329]
        tunnel: [w328] -> w253
        i -> [w331]
        stop <- w332 stop-if-true
        n192 = Increment(x=w331) -> (x+1=w334:i32)
        n193 = Wait (ms)(milliseconds to wait=u32 50) -> ()  [unwired: 1 out]
        n194 = Greater Or Equal?(x=w334, y=40) -> (x >= y?=w332:bool)
        n195 = call <vilib>:"WPI_MotorControlSetOutput.vi"("Output"=-0.2, "MotorControlDevRef"=w329) -> ("MotorControlDevRef"=w328:T3)  [unwired: 7 in, 2 out]
      }
      n196 = while {
        tunnel: w262 -> [w363]
        tunnel: w261 -> [w362]
        tunnel: [w361] -> w260
        tunnel: [w360] -> w259
        i -> [w366]
        stop <- w367 stop-if-true
        w365 = FALSE
        n197 = Increment(x=w366) -> (x+1=w369:i32)
        n198 = Not(x=w365) -> (.not. x?=w364:bool)
        n199 = Wait (ms)(milliseconds to wait=u32 50) -> ()  [unwired: 1 out]
        n200 = Greater Or Equal?(x=w369, y=65) -> (x >= y?=w367:bool)
        n201 = call-poly <vilib>:"WPI_SolenoidSet.vi"("Value"=w365, "SolenoidDevRef"=w362) -> ("SolenoidDevRef"=w360:T7)  [unwired: 8 in, 1 out]
        n202 = call-poly <vilib>:"WPI_SolenoidSet.vi"("Value"=w364, "SolenoidDevRef"=w363) -> ("SolenoidDevRef"=w361:T7)  [unwired: 8 in, 1 out]
      }
      n203 = while {
        tunnel: w272 -> [w412]
        tunnel: [w404] -> w263
        i -> [w406]
        stop <- w407 stop-if-true
        n204 = Increment(x=w406) -> (x+1=w409:i32)
        n205 = Wait (ms)(milliseconds to wait=u32 50) -> ()  [unwired: 1 out]
        n206 = call-poly <vilib>:"WPI_RobotDriveArcadeDrive.vi"("Y axis value"=0.0 ("X axis value"), "X axis value"=0.5, "RobotDriveDevRef"=w412) -> ("RobotDriveDevRef"=w404:T9)  [unwired: 6 in, 2 out]
        n207 = Greater Or Equal?(x=w409, y=65) -> (x >= y?=w407:bool)
      }
      n208 = while {
        tunnel: w253 -> [w302]
        tunnel: [w301] -> w252
        i -> [w304]
        stop <- w305 stop-if-true
        n209 = Increment(x=w304) -> (x+1=w307:i32)
        n210 = call <vilib>:"WPI_MotorControlSetOutput.vi"("Output"=-0.2, "MotorControlDevRef"=w302) -> ("MotorControlDevRef"=w301:T3)  [unwired: 7 in, 2 out]
        n211 = Wait (ms)(milliseconds to wait=u32 50) -> ()  [unwired: 1 out]
        n212 = Greater Or Equal?(x=w307, y=65) -> (x >= y?=w305:bool)
      }
      n213 = while {
        tunnel: w260 -> [w312]
        tunnel: w259 -> [w311]
        tunnel: [w310] -> w250
        tunnel: [w309] -> w249
        i -> [w315]
        stop <- w316 stop-if-true
        w314 = FALSE
        n214 = Increment(x=w315) -> (x+1=w318:i32)
        n215 = Not(x=w314) -> (.not. x?=w313:bool)
        n216 = Wait (ms)(milliseconds to wait=u32 50) -> ()  [unwired: 1 out]
        n217 = Greater Or Equal?(x=w318, y=10) -> (x >= y?=w316:bool)
        n218 = call-poly <vilib>:"WPI_SolenoidSet.vi"("Value"=w314, "SolenoidDevRef"=w311) -> ("SolenoidDevRef"=w309:T7)  [unwired: 8 in, 1 out]
        n219 = call-poly <vilib>:"WPI_SolenoidSet.vi"("Value"=w313, "SolenoidDevRef"=w312) -> ("SolenoidDevRef"=w310:T7)  [unwired: 8 in, 1 out]
      }
      n220 = while {
        tunnel: w263 -> [w327]
        i -> [w321]
        stop <- w322 stop-if-true
        n221 = Increment(x=w321) -> (x+1=w324:i32)
        n222 = Wait (ms)(milliseconds to wait=u32 50) -> ()  [unwired: 1 out]
        n223 = call-poly <vilib>:"WPI_RobotDriveArcadeDrive.vi"("Y axis value"=0.0 ("X axis value"), "X axis value"=0.0, "RobotDriveDevRef"=w327) -> ()  [unwired: 6 in, 3 out]
        n224 = Greater Or Equal?(x=w324, y=10) -> (x >= y?=w322:bool)
      }
      n225 = while {
        tunnel: w252 -> [w294]
        tunnel: [w293] -> w251
        i -> [w296]
        stop <- w297 stop-if-true
        n226 = Increment(x=w296) -> (x+1=w299:i32)
        n227 = Wait (ms)(milliseconds to wait=u32 50) -> ()  [unwired: 1 out]
        n228 = call <vilib>:"WPI_MotorControlSetOutput.vi"("Output"=1.0, "MotorControlDevRef"=w294) -> ("MotorControlDevRef"=w293:T3)  [unwired: 7 in, 2 out]
        n229 = Greater Or Equal?(x=w299, y=5) -> (x >= y?=w297:bool)
      }
      n230 = while {
        tunnel: w250 -> [w278]
        tunnel: w249 -> [w277]
        i -> [w281]
        stop <- w282 stop-if-true
        w280 = TRUE
        n231 = Increment(x=w281) -> (x+1=w284:i32)
        n232 = Not(x=w280) -> (.not. x?=w279:bool)
        n233 = Wait (ms)(milliseconds to wait=u32 50) -> ()  [unwired: 1 out]
        n234 = Greater Or Equal?(x=w284, y=5) -> (x >= y?=w282:bool)
        n235 = call-poly <vilib>:"WPI_SolenoidSet.vi"("Value"=w280, "SolenoidDevRef"=w277) -> ()  [unwired: 8 in, 2 out]
        n236 = call-poly <vilib>:"WPI_SolenoidSet.vi"("Value"=w279, "SolenoidDevRef"=w278) -> ()  [unwired: 8 in, 2 out]
      }
      n237 = while {
        tunnel: w251 -> [w286]
        i -> [w288]
        stop <- w289 stop-if-true
        n238 = Increment(x=w288) -> (x+1=w291:i32)
        n239 = Wait (ms)(milliseconds to wait=u32 50) -> ()  [unwired: 1 out]
        n240 = call <vilib>:"WPI_MotorControlSetOutput.vi"("Output"=0.0, "MotorControlDevRef"=w286) -> ()  [unwired: 7 in, 3 out]
        n241 = Greater Or Equal?(x=w291, y=5) -> (x >= y?=w289:bool)
      }
    }
    frame 0, Default {
    }
  }
  n242 = while {
    stop <- FALSE stop-if-true
    n243 = call <vilib>:"WPI_DriverStationReport Robot Code State.vi"("Autonomous"=TRUE) -> ()  [unwired: 10 in, 1 out]
    n244 = Wait (ms)(milliseconds to wait=u32 20) -> ()  [unwired: 1 out]
  }
  n245 = call <vilib>:"WPI_JoystickRefNum Registry Get.vi"("refnum name"="Joystick 0") -> ("JoystickDevRef"=w8:T10)  [unwired: 1 in, 9 out]
  n246 = call <vilib>:"WPI_JoystickGetValues.vi"("JoystickDevRef"=w8) -> ("Axes"=w6:dbl[])  [unwired: 6 in, 4 out]
  n247 = call <vilib>:"SD Write Numeric Array.vi"("Numeric Array"=w6, "Name"="Joystick 0/Axes") -> ()  [unwired: 8 in, 2 out]
  n248 = call <vilib>:"WPI_RobotDriveRefNum Registry Get.vi"("refnum name"="Left and Right Motors") -> ("RobotDriveDevRef"=w4:T9)  [unwired: 1 in, 9 out]
  n249 = for {
    shift-right: [w447] -> _
    shift-left: w4 -> [w448]
    tunnel: "Array of robot movements" -> [w443] mode=indexing
    n250 = Unbundle By Name(w443) -> ("X Joystick Value"=w446:dbl, "Y Joystick Value"=w445:dbl, "Delay (sec)"=w444:dbl)  [unwired: 1 out]
    n251 = call-poly <vilib>:"WPI_RobotDriveArcadeDrive.vi"("Y axis value"=w445, "X axis value"=w446, "RobotDriveDevRef"=w448) -> ("Motor Values"=w442:dbl[], "RobotDriveDevRef"=w449:T9)  [unwired: 1 in, 6 out]
    n252 = call-poly <vilib>:"SD Write Value.vi"("Numeric Array"=w442, "Name"="RobotDrive Motors") -> ()  [unwired: 8 in, 2 out]
    n253 = call <vilib>:"WPI_RobotDriveDelayAndUpdateSafety.vi"("Delay (s)"=w444, "RobotDriveDevRef"=w449) -> ("RobotDriveDevRef 2"=w447:T9)  [unwired: 8 in, 1 out]
    "Current Movement, for debugging" <- w443
  }
